vi "Log Data.vi"(8 "error in (no error)":errorcluster, 10 "Data Queue":refnum<queue>, 11 "Logging Configuration":T1) -> (0 "error out":errorcluster, 3 "Data Log Refnum":refnum<k1>)   [LabVIEW 2018, in "Logging.lvlib"]
doc: "Use the Write To Measurement File Express VI to log data to disk in a LVM file."
uses:
  Logging.lvlib
  Logging Configuration.ctl
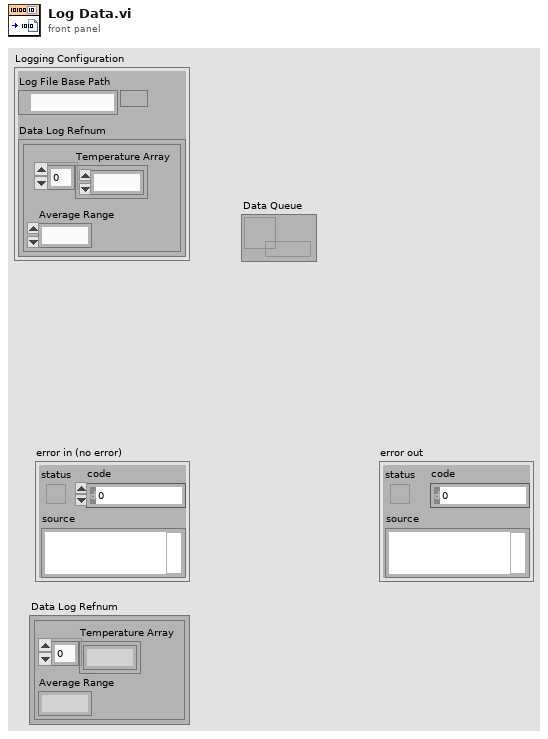
[diagram p1: front panel]
types:
  T1 = typedef "Logging.lvlib/Logging Configuration.ctl" = cluster{"Log File Base Path":path, "Data Log Refnum":refnum<k1>}
  T2 = cluster{"Temperature Array":dbl[], "Average Range":dbl}
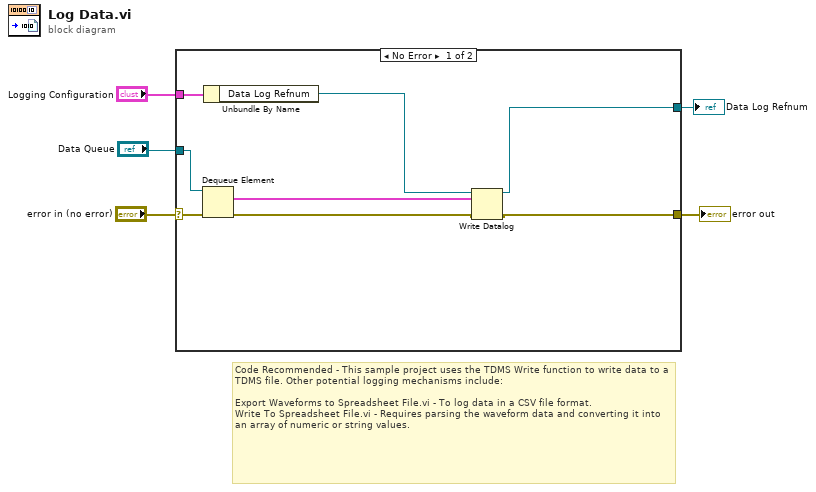
[diagram p0: block diagram]
diagram:
  # "Code Recommended - This sample project uses the TDMS Write function to write data to a TDMS file. Other potential logging mechanisms include:\n\nExport Waveforms to Spreadsheet File.vi - To log data in a CSV file format.\nWrite To Spreadsheet File.vi - Requires parsing the waveform data and converting it into an array of numeric or string values."
  n1 = case shown="No Error" "error in (no error)" {
    selector: "error in (no error)" -> [w13 w14]
    tunnel: "Logging Configuration" -> [w7 _]
    tunnel: "Data Queue" -> [w12 _]
    tunnel: [w11 w14] -> w5
    tunnel: [w9 _] -> w1
    frame No Error {
      n2 = Dequeue Element(queue=w12, error in (no error)=w13) -> (element=w6:T2, error out=w10:errorcluster)  [unwired: 1 in, 2 out]
      n3 = Unbundle By Name(w7) -> ("Data Log Refnum"=w8:refnum<k1>)
      n4 = Write Datalog(4:w10, 6:w6, 7:w8) -> (0:w11:errorcluster, 3:w9:refnum<k1>)
    }
    frame Error {
    }
  }
  "error out" <- w5
  "Data Log Refnum" <- w1
